vi "Connect.vi"(8 "error in":errorcluster, 11 "79XRP in":refnum<class "79XRP.lvclass">) -> (0 "error out":errorcluster, 3 "79XRP out":refnum<class "79XRP.lvclass">)   [LabVIEW 2019, in "79XRP.lvlib" / "79XRP.lvclass"]
uses:
  Library/79XRP.lvclass
  C:/Users/Public/Documents/Development/builds/Instruments/Instruments.lvlibp/Library/Instruments.lvclass
  C:/Users/Public/Documents/Development/builds/Instruments/PowerSupply.lvlibp/Library/PowerSupply.lvclass
  Library/79XRP.lvclass/79XRP.ctl
  builds/Instruments/Instruments.lvlibp/Accessors/Read Resource.vi
  Accessors/Read Local Resource.vi
  Accessors/Write Local Resource.vi
  <instrlib>/Keysight RP7900 Series/Keysight RP7900 Series.lvlib
  builds/Engine/Engine.lvlibp/Project/Engine.lvclass
  C:/Users/Public/Documents/Development/builds/Engine/Engine.lvlibp/Project/Engine.lvclass
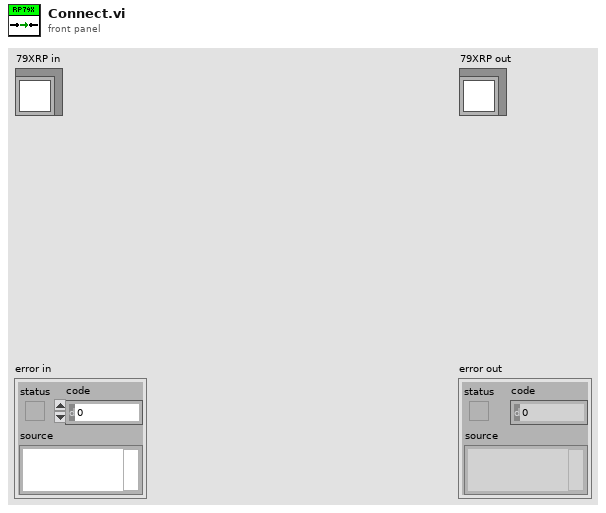
[diagram p1: front panel]
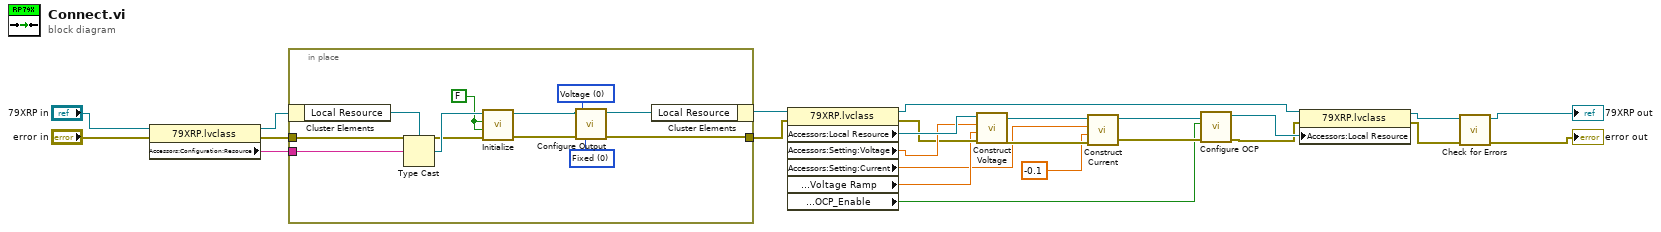
[diagram p0: block diagram]
diagram:
  n1 = property class="79XRP.lvclass"(reference="79XRP in", error in="error in") -> (reference out=w23:refnum<class "79XRP.lvclass">, error out=w22:errorcluster, "Accessors:Configuration:Resource"=w24:string)
  n2 = in-place {
    in-place-border: w24 -> [w35]
    in-place-border: w22 -> [w32]
    in-place-border: [w26] -> w16
    w28 = u16 0 items=["Fixed", "Step", "List", "Arbitrary"] ("Output Transient Mode (0: Fixed)")
    w29 = u16 0 items=["Voltage", "Current"] ("Output Priority Mode (0: Voltage)")
    w33 = FALSE ("ID Query (True)")
    n3 = in-place-cluster #1(w23) -> ("Local Resource"=w36:refnum<visa-resource-name>)
    n4 = Type Cast(type=w36, x=w35) -> (*(type *) &x=w34:refnum<visa-resource-name>)
    n5 = call <instrlib>:"Initialize.vi"("error in (no error)"=w32, "Reset (True)"=w33, "ID Query (True)"=w33, "VISA resource name"=w34) -> ("error out"=w30:errorcluster, "VISA resource name out"=w31:refnum<visa-resource-name>)  [unwired: 6 in]
    n6 = call <instrlib>:"Configure Output.vi"("error in (no error)"=w30, "Output Transient Mode (0: Fixed)"=w28, "Output Priority Mode (0: Voltage)"=w29, "VISA resource name"=w31) -> ("error out"=w26:errorcluster, "VISA resource name out"=w27:refnum<visa-resource-name>)  [unwired: 6 in]
    n7 = in-place-cluster #1("Local Resource"=w27) -> (w20:refnum<class "79XRP.lvclass">)
  }
  n8 = property class="79XRP.lvclass"(reference=w20, error in=w16) -> (reference out=w19:refnum<class "79XRP.lvclass">, error out=w13:errorcluster, "Accessors:Local Resource"=w15:refnum<visa-resource-name>, "Accessors:Setting:Voltage"=w14:dbl, "Accessors:Setting:Current"=w2:dbl, "Accessors:Setting:Ramp:Voltage Ramp"=w8:dbl, "Accessors:Setting:Protection:OCP_Enable"=w1:bool)
  n9 = call "Construct Voltage.vi"("error in (no error)"=w13, "Slew"=w8, "Voltage"=w14, "VISA resource name"=w15) -> ("error out"=w4:errorcluster, "VISA resource name out"=w7:refnum<visa-resource-name>)  [unwired: 6 in]
  n10 = call "Construct Current.vi"("error in (no error)"=w4, "Negative Current Limit"=-0.1 ("Voltage Priority Current Lower Limit (0 A)"), "Positive Current Limit"=w2, "VISA resource name"=w7) -> ("error out"=w5:errorcluster, "VISA resource name out"=w6:refnum<visa-resource-name>)  [unwired: 6 in]
  n11 = call <instrlib>:"Configure OCP.vi"("error in (no error)"=w5, "Enable OCP (F: Disable)"=w1, "VISA resource name"=w6) -> ("error out"=w17:errorcluster, "VISA resource name out"=w18:refnum<visa-resource-name>)  [unwired: 7 in]
  n12 = property class="79XRP.lvclass"(reference=w19, error in=w17, "Accessors:Local Resource"=w18) -> (reference out=w12:refnum<class "79XRP.lvclass">, error out=w9:errorcluster)
  n13 = call "Check for Errors.vi"("error in"=w9, "Engine in"=w12) -> ("error out"=→"error out":errorcluster, "Engine out"=→"79XRP out":refnum<class "79XRP.lvclass">)  [unwired: 8 in]
